vi "Get Elements On Board.vi"(11 "Board Game in":refnum<class "Board Game.lvclass">) -> (2 "Color Array":T1(array[cluster]), 3 "position":cluster{"x":dbl, "y":dbl}[](array[cluster]))   [LabVIEW 2021, in "Board Game.lvclass"]
uses:
  Board Game.lvclass
  Board Game.lvclass/Board Game.ctl
  GameEl_class/GameEl.lvclass/GameEl.ctl
  GameEl_class/Read Colour.vi
  GameEl_class/Read position.vi
  GameEl_class/Read Visible.vi
  Snake_class/Snake.lvclass
  C:/Users/poche/Programs/LabVIEW/imposible snake/GameEl_class/GameEl.lvclass
  Fruit_class/Fruit.lvclass
  Bomb/Bomb.lvclass
  Shield/Shield.lvclass
  Grape/Grape.lvclass
  Mouse/Mouse.lvclass
  Cricket/Cricket.lvclass
  Star/Star.lvclass
  GameEl_class/GameEl.lvclass
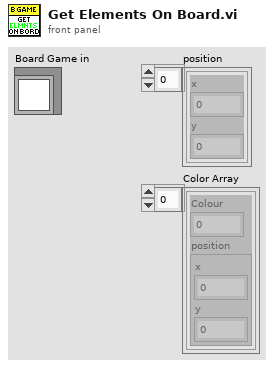
[diagram p1: front panel]
types:
  T1 = cluster{"Colour":u32, "position":cluster{"x":dbl, "y":dbl}}[]
  T2 = cluster{"SubVIs:DataAccess:Colour":u32, "position":cluster{"x":dbl, "y":dbl}}
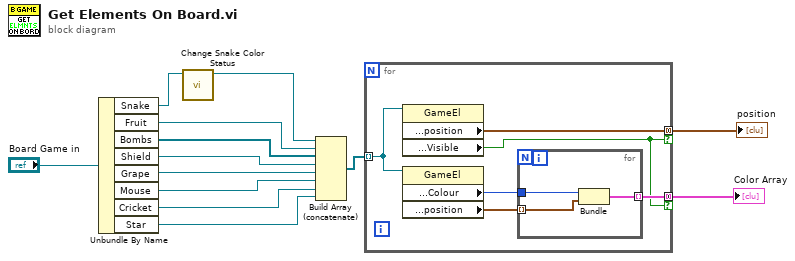
[diagram p0: block diagram]
diagram:
  n1 = Unbundle By Name("Board Game in") -> ("Snake"=w6:refnum<class "Snake.lvclass">, "Fruit"=w4:refnum<class "Fruit.lvclass">, "Bombs"=w9:refnum<class "Bomb.lvclass">[], "Shield"=w10:refnum<class "Shield.lvclass">, "Grape"=w11:refnum<class "Grape.lvclass">, "Mouse"=w3:refnum<class "Mouse.lvclass">, "Cricket"=w2:refnum<class "Cricket.lvclass">, "Star"=w1:refnum<class "Star.lvclass">)
  n2 = call "Change Snake Color Status.vi"("Snake in"=w6) -> ("Snake out"=w5:refnum<class "Snake.lvclass">)  [unwired: 9 in, 1 out]
  n3 = Build Array (concatenate)(w5, w4, w9, w10, w11, w3, w2, w1) -> (w12:refnum<class "GameEl.lvclass">[])
  n4 = for {
    tunnel: w12 -> [w18] mode=indexing
    tunnel: [w19] -> w13 mode=concatenating if=w14
    tunnel: [w15] -> w7 mode=concatenating if=w14
    n5 = property class="GameEl"(reference=w18) -> ("SubVIs:DataAccess:position"=w19:cluster{"x":dbl, "y":dbl}[], "SubVIs:DataAccess:Visible"=w14:bool)  [unwired: 1 in, 2 out]
    n6 = property class="GameEl"(reference=w18) -> ("SubVIs:DataAccess:Colour"=w17:u32, "SubVIs:DataAccess:position"=w16:cluster{"x":dbl, "y":dbl}[])  [unwired: 1 in, 2 out]
    n7 = for {
      tunnel: w17 -> [w21]
      tunnel: w16 -> [w22] mode=indexing
      tunnel: [w20] -> w15 mode=indexing
      n8 = Bundle("SubVIs:DataAccess:Colour"=w21, "position"=w22) -> (w20:T2)  [unwired: 1 in]
    }
  }
  "position" <- w13
  "Color Array" <- w7
